vi "WrapSignal.vi"(3 "DataIn":dbl[](array[numeric])) -> (1 "SmoothWrappedData":dbl[](array[numeric]))   [LabVIEW 2022 SP3]
uses:
  <vilib>/gmath/NI_Gmath.lvlib
panel:
  out "WrapRegion":cluster{"xi":dbl[], "yi":dbl[]}[](graph)
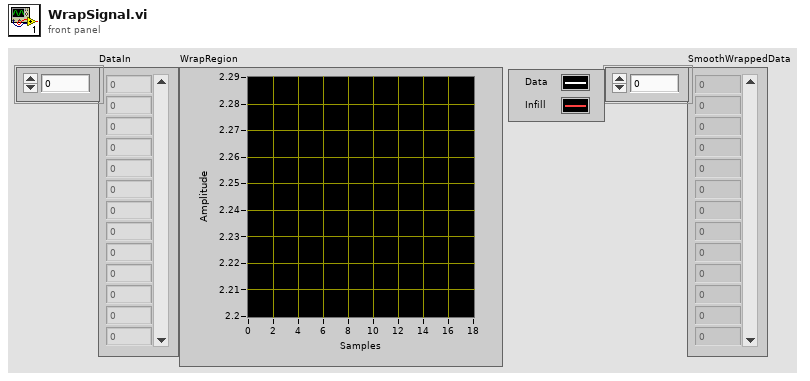
[diagram p1: front panel]
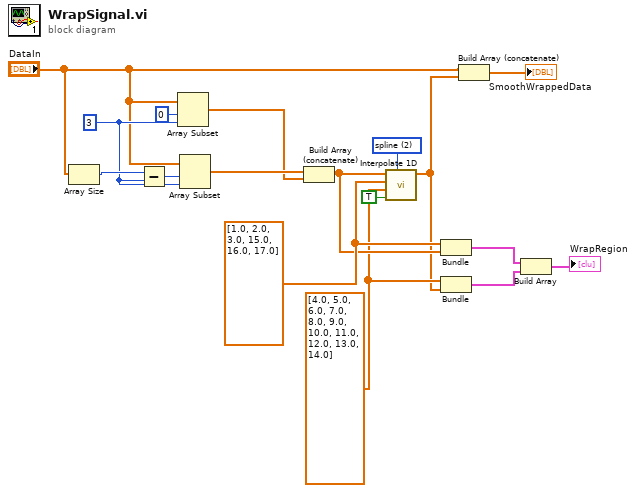
[diagram p0: block diagram]
diagram:
  w10 = 2 items=["nearest", "linear", "spline", "cubic Hermite", "Lagrange"] ("method")
  w7 = dbl[] [4.0, 5.0, 6.0, 7.0, 8.0, 9.0, 10.0, 11.0, 12.0, 13.0, 14.0] ("xi")
  w9 = dbl[] [1.0, 2.0, 3.0, 15.0, 16.0, 17.0] ("X")
  w14 = 3 ("length")
  n1 = Array Size(array="DataIn") -> (size(s)=w16:i32)
  n2 = Subtract(x=w16, y=w14) -> (x-y=w15:i32)
  n3 = Array Subset(array="DataIn", index=0, length=w14) -> (w12:dbl[])
  n4 = Array Subset(array="DataIn", index=w15, length=w14) -> (w13:dbl[])
  n5 = Build Array (concatenate)(w13, w12) -> (w8:dbl[])
  n6 = call <vilib>:"Interpolate 1D.vi"("method"=w10, "X is monotonic"=TRUE, "xi"=w7, "X"=w9, "Y"=w8) -> ("yi"=w2:dbl[])  [unwired: 4 in, 2 out]
  n7 = Bundle("X"=w9, w8) -> (w5:cluster{"X":dbl[], dbl[]})  [unwired: 1 in]
  n8 = Bundle("xi"=w7, "yi"=w2) -> (w6:cluster{"xi":dbl[], "yi":dbl[]})  [unwired: 1 in]
  n9 = Build Array (concatenate)("DataIn", w2) -> (→"SmoothWrappedData":dbl[])
  n10 = Build Array(w5, w6) -> (→"WrapRegion":cluster{"xi":dbl[], "yi":dbl[]}[])
